vi "Read connection counter.vi"(8 "error in (no error)":errorcluster, 11 "TCP Slave in":refnum<class "TCP Server.lvclass">) -> (0 "error out":errorcluster, 2 "Currently Connected":u32, 3 "TCP Slave out":refnum<class "TCP Server.lvclass">)   [LabVIEW 2021, in "WebSockets.lvlib" / "TCP Server.lvclass"]
uses:
  TCP Server.lvclass
  TCP Server.lvclass/TCP Server.ctl
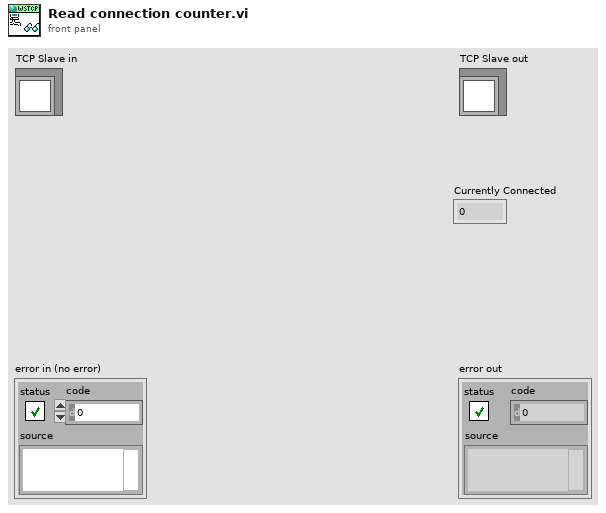
[diagram p1: front panel]
types:
  T1 = typedef "WebSockets.lvlib/TCP Server.lvclass/Connection Counter.ctl" = cluster{"Currently Connected":u32, "Connection Records":refnum<data-value>[]}
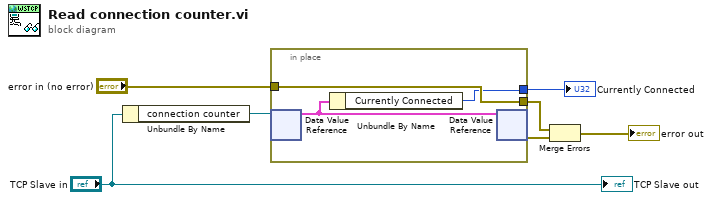
[diagram p0: block diagram]
diagram:
  n1 = Unbundle By Name("TCP Slave in") -> ("connection counter"=w2:refnum<data-value>)
  n2 = in-place {
    in-place-border: "error in (no error)" -> [w10]
    in-place-border: [w10] -> w5
    in-place-border: [w8] -> w1
    n3 = in-place-dvr #1(w2) -> (w9:T1)  [unwired: 1 out]
    n4 = Unbundle By Name(w9) -> ("Currently Connected"=w8:u32)
    n5 = in-place-dvr #1(w9) -> (w6:errorcluster)  [unwired: 1 out]
  }
  "Currently Connected" <- w1
  n6 = Merge Errors(w5, w6) -> (→"error out":errorcluster)
  "TCP Slave out" <- "TCP Slave in"
